vi "mainFPGA.vi"(11 "waitInMs":u32) -> (3 "dataFifoFull":bool)   [LabVIEW 2018]
doc: "Read analog sensors and relays status from NI modules. Put this data into the <b>daqFIFO</b>."
uses:
  <vilib>/rvi/Emulation/niFpgaGetClockAttributes.vi
  <vilib>/rvi/Emulation/niFpgaSctlEmulationGetInTimedLoop.vi
  <vilib>/rvi/Emulation/niFpgaEmulationReportErrorSimple.vi
  <vilib>/rvi/interface/RandomDataEmulation/niFpgaRandomDataHandleErrors.vi
  <vilib>/rvi/Emulation/niFpgaCriticalErrorInLSC.vi
  <vilib>/rvi/DataTransferAndStorage/Container/XNode/niFpgaContainer.xnode
  <vilib>/rvi/interface/RandomDataEmulation/nirviRandomDataFpgaReadWriteTemplate.vi
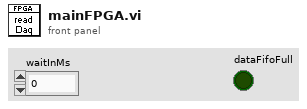
[diagram p1: front panel]
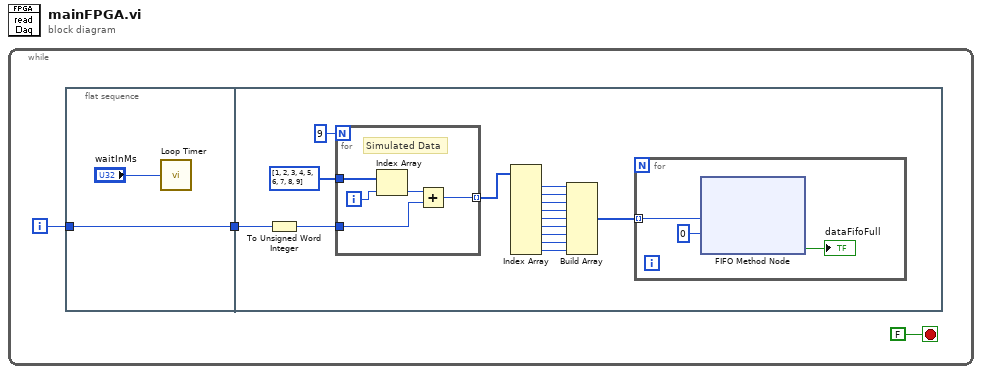
[diagram p0: block diagram]
diagram:
  n1 = while {
    i -> [w1]
    stop <- FALSE stop-if-true
    n2 = flat-sequence {
      tunnel: [w4] -> w2
      tunnel: w1 -> [w4]
      tunnel: w2 -> [w7]
      frame #0 {
        n3 = call "Loop Timer"("Count(mSec)"="waitInMs") -> ()  [unwired: 1 out]
      }
      frame #1 {
        n4 = To Unsigned Word Integer(number=w7) -> (unsigned 16bit integer=w6:u16)
        n5 = for {
          N: 9 -> [_]
          tunnel: u16[] [1, 2, 3, 4, 5, 6, 7, 8, 9] -> [w25]
          tunnel: w6 -> [w22]
          tunnel: [w21] -> w10 mode=indexing
          i -> [w24]
          # "Simulated Data"
          n6 = Index Array(array=w25, index=w24) -> (element=w23:u16)
          n7 = Add(x=w23, y=w22) -> (x+y=w21:u16)
        }
        n8 = Index Array(array=w10) -> (element #1=w14:u16, element #2=w13:u16, element #3=w12:u16, element #4=w11:u16, element #5=w20:u16, element #6=w19:u16, element #7=w18:u16, element #8=w17:u16, element #9=w16:u16)  [unwired: 9 in]
        n9 = Build Array(w14, w13, w12, w11, w20, w19, w18, w17, w16) -> (w15:u16[])
        n10 = for {
          tunnel: w15 -> [w27] mode=indexing
          n11 = xnode ("FIFO Method Node")("Element"=w27, "Timeout"=0) -> ("Timed Out?"=→"dataFifoFull":bool)  [unwired: 1 in, 1 out]
        }
      }
    }
  }
